vi "readFromXML.vi"(8 "error in (no error)":errorcluster, 10 "XML in":string, 11 "CommandsForAzElAxes in":refnum<class "CommandsForAzElAxes.lvclass">) -> (0 "error out":errorcluster, 3 "CommandsForAzElAxes out":refnum<class "CommandsForAzElAxes.lvclass">)   [LabVIEW 2022 SP3, in "TCSDataDefinitions.lvlib" / "TCSMountControlCommand.lvlib" / "CommandsForAzElAxes.lvlib" / "CommandsForAzElAxes.lvclass"]
uses:
  CommandsForAzElAxes.lvclass
  TCSMCCCommand/TCSMCCCommand.lvclass
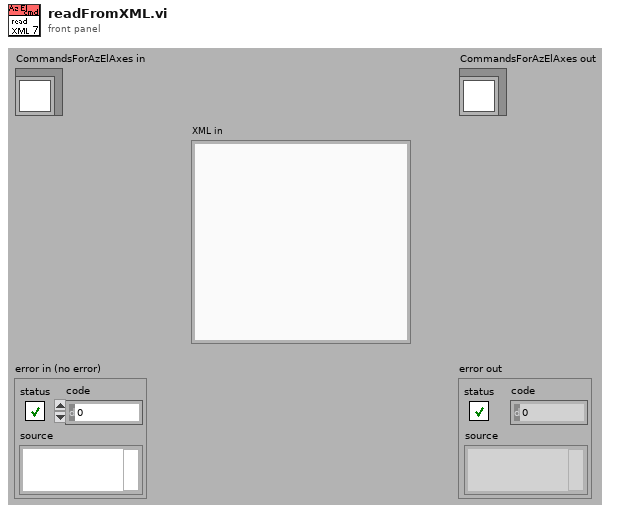
[diagram p1: front panel]
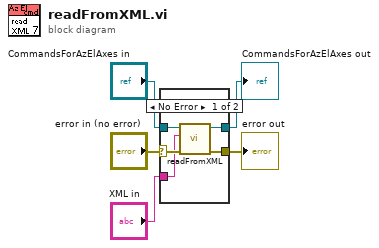
[diagram p0: block diagram]
diagram:
  n1 = case shown="No Error" "error in (no error)" {
    selector: "error in (no error)" -> [w8 w12]
    tunnel: [w6 w12] -> w4
    tunnel: [w9 w11] -> w2
    tunnel: "CommandsForAzElAxes in" -> [w10 w11]
    tunnel: "XML in" -> [w7 _]
    frame No Error {
      n2 = call-parent "readFromXML.vi"("error in (no error)"=w8, "XML in"=w7, "TCSMCCCommand in"=w10) -> ("error out"=w6:errorcluster, "TCSMCCCommand out"=w9:refnum<class "CommandsForAzElAxes.lvclass">)  [unwired: 7 out]
    }
    frame Error {
    }
  }
  "error out" <- w4
  "CommandsForAzElAxes out" <- w2
